vi "Load Patterns to Sessions.vi"(8 "error in":errorcluster, 10 "Pattern file paths":string[](array[string]), 11 "Sequence Context":refnum<k7>) -> (0 "error out":errorcluster)   [LabVIEW 2020, in "NIDigitalSPI.lvlib"]
uses:
  NIDigitalSPI.lvlib
  <vilib>/MeasurementLink/MeasurementLink Session Management Client/RPC Messages/ni_measurementlink_sessionmanagement_v1_ReserveSessionsRequest.ctl
  <vilib>/MeasurementLink/MeasurementLink Session Management Client/RPC Messages/ni_measurementlink_PinMapContext.ctl
  <vilib>/MeasurementLink/MeasurementLink Discovery Client/RPC Messages/ni_measurementlink_discovery_v1_ResolveServiceRequest.ctl
  <instrlib>/niDigital/niDigital.llb/niDigital gRPC Device Server.ctl
  <vilib>/MeasurementLink/MeasurementLink Session Management Client/MeasurementLink Session Management Client.lvlib
  <vilib>/MeasurementLink/MeasurementLink Discovery Client/MeasurementLink Discovery Client.lvlib
  <vilib>/MeasurementLink/MeasurementLink Measurement Server/MeasurementLink Measurement Server.lvlib
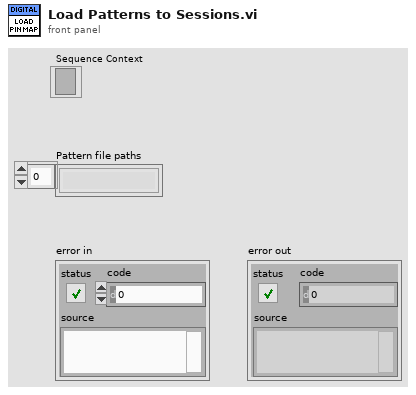
[diagram p1: front panel]
types:
  T1 = typedef "MeasurementLink Discovery Client.lvlib/ni_measurementlink_discovery_v1_ResolveServiceRequest.ctl" = cluster{"provided_interface":string, "service_class":string}
  T2 = typedef "MeasurementLink Session Management Client.lvlib/ni_measurementlink_sessionmanagement_v1_ReserveSessionsRequest.ctl" = cluster{"pin_map_context":T3, "pin_or_relay_names":string[], "instrument_type_id":string, "timeout_in_milliseconds":i32}
  T3 = typedef "MeasurementLink Session Management Client.lvlib/ni_measurementlink_PinMapContext.ctl" = cluster{"pin_map_id":string, "sites":i32[]}
  T4 = typedef "grpc-lvsupport-release.lvlib/grpcId.ctl" = u64
  T5 = typedef "MeasurementLink Discovery Client.lvlib/ni_measurementlink_discovery_v1_ServiceLocation.ctl" = cluster{"location":string, "insecure_port":string, "ssl_authenticated_port":string}
  T6 = typedef "MeasurementLink Session Management Client.lvlib/ni_measurementlink_sessionmanagement_v1_ReserveSessionsResponse.ctl" = cluster{"sessions":T7[]}
  T7 = typedef "MeasurementLink Session Management Client.lvlib/ni_measurementlink_sessionmanagement_v1_SessionInformation.ctl" = cluster{"session":T8, "resource_name":string, "channel_list":string, "instrument_type_id":string, "session_exists":bool, "channel_mappings":T9[]}
  T8 = typedef "MeasurementLink Session Management Client.lvlib/nidevice_grpc_Session.ctl" = cluster{"name":string}
  T9 = typedef "MeasurementLink Session Management Client.lvlib/ni_measurementlink_sessionmanagement_v1_ChannelMapping.ctl" = cluster{"pin_or_relay_name":string, "site":i32, "channel":string}
  T10 = typedef "niDigital gRPC Device Server.ctl" = cluster{"session name":string, "address (localhost)":string, "port (31763)":u32}
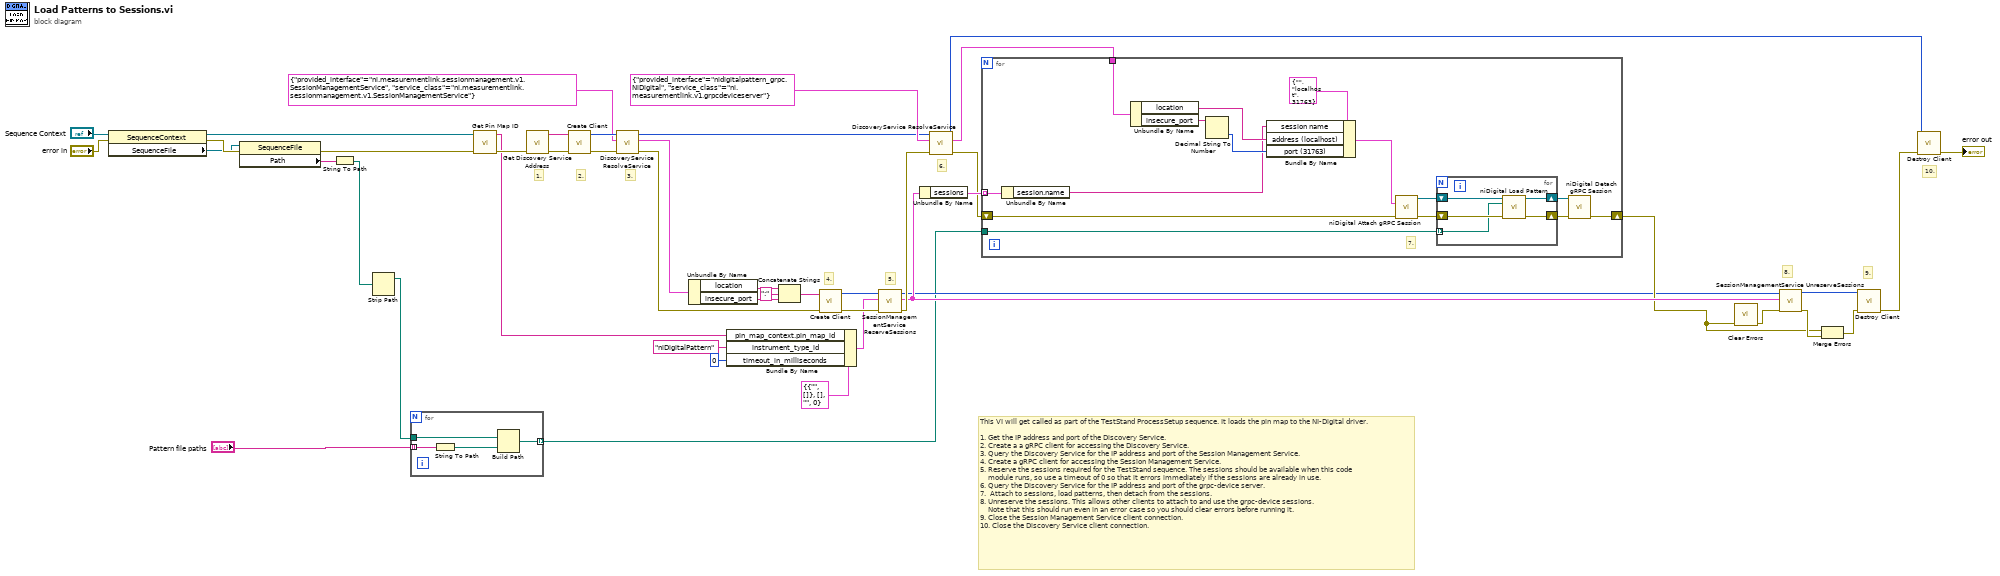
[diagram p0: block diagram]
diagram:
  # "10."
  # "9."
  # "8."
  # "6."
  # "5."
  # "4."
  # "3."
  # "2."
  # "1."
  # "This VI will get called as part of the TestStand ProcessSetup sequence. It loads the pin map to the NI-Digital driver.\n\n1. Get the IP address and port of the Discovery Service.\n2. Create a a gRPC client for accessing the Discovery Service.\n3. Query the Discovery Service for the IP address and port of the Session Management Service.\n4. Create a gRPC client for accessing the Session Management Service.\n5. Reserve the sessions required for the TestStand sequence. The sessions should be available when this code\n    module runs, so use a timeout of 0 so that it errors immediately if the sessions are already in use.  \n6. Query the Discovery Service for the IP address and port of the grpc-device server.\n7.  Attach to sessions, load patterns, then detach from the sessions.\n8. Unreserve the sessions. This allows other clients to attach to and use the grpc-device sessions. \n    Note that this should run even in an error case so you should clear errors before running it.\n9. Close the Session Management Service client connection.\n10. Close the Discovery Service client connection."
  n1 = property class="SequenceContext"(reference="Sequence Context", error in="error in") -> (reference out=w6:refnum<k7>, error out=w11:errorcluster, "SequenceFile"=w10:refnum<k7>)
  n2 = property class="SequenceFile"(reference=w10, error in=w11) -> (error out=w5:errorcluster, "Path"=w9:string)  [unwired: 1 out]
  n3 = String To Path(string=w9) -> (path=w4:path)
  n4 = Strip Path(path=w4) -> (stripped path=w2:path)  [unwired: 1 out]
  n5 = for {
    tunnel: "Pattern file paths" -> [w50] mode=indexing
    tunnel: [w47] -> w1 mode=indexing
    tunnel: w2 -> [w49]
    n6 = String To Path(string=w50) -> (path=w48:path)
    n7 = Build Path(base path=w49, name or relative path=w48) -> (appended path=w47:path)
  }
  n8 = call "Get Pin Map ID.vi"("error in"=w5, "Sequence Context"=w6) -> ("error out"=w20:errorcluster, "pin_map_id"=w19:string)  [unwired: 8 in]
  n9 = call <vilib>:"Get Discovery Service Address.vi"("error in"=w20) -> ("error out"=w27:errorcluster, "address"=w26:string)  [unwired: 9 in]
  n10 = call <vilib>:"Create Client.vi"("error in"=w27, "address"=w26) -> ("error out"=w43:errorcluster, "gRPC ID Out"=w44:T4)  [unwired: 8 in]
  n11 = call <vilib>:"DiscoveryService ResolveService.vi"("error in"=w43, "Request Data"=T1 {"provided_interface"="ni.measurementlink.sessionmanagement.v1.SessionManagementService", "service_class"="ni.measurementlink.sessionmanagement.v1.SessionManagementService"}, "gRPC ID"=w44) -> ("error out"=w42:errorcluster, "Response Data"=w14:T5, "gRPC ID out"=w33:T4)  [unwired: 6 in]
  n12 = Unbundle By Name(w14) -> ("location"=w16:string, "insecure_port"=w17:string)
  n13 = Bundle By Name(cluster=T2 {"pin_map_context"={"pin_map_id"="", "sites"=[]}, "pin_or_relay_names"=[], "instrument_type_id"="", "timeout_in_milliseconds"=0} ("Request Data"), "pin_map_context.pin_map_id"=w19, "instrument_type_id"="niDigitalPattern", "timeout_in_milliseconds"=0) -> (w38:T2)
  n14 = Concatenate Strings(w16, ":" ("string"), w17) -> (w15:string)
  n15 = call <vilib>:"Create Client.vi"("error in"=w42, "address"=w15) -> ("error out"=w45:errorcluster, "gRPC ID Out"=w46:T4)  [unwired: 8 in]
  n16 = call <vilib>:"SessionManagementService ReserveSessions.vi"("error in"=w45, "Request Data"=w38, "gRPC ID"=w46) -> ("error out"=w31:errorcluster, "Response Data"=w22:T6, "gRPC ID out"=w12:T4)  [unwired: 6 in]
  n17 = Unbundle By Name(w22) -> ("sessions"=w35:T7[])
  n18 = call <vilib>:"DiscoveryService ResolveService.vi"("error in"=w31, "Request Data"=T1 {"provided_interface"="nidigitalpattern_grpc.NiDigital", "service_class"="ni.measurementlink.v1.grpcdeviceserver"}, "gRPC ID"=w33) -> ("error out"=w30:errorcluster, "Response Data"=w29:T5, "gRPC ID out"=w32:T4)  [unwired: 6 in]
  n19 = for {
    tunnel: w35 -> [w64] mode=indexing
    shift-right: [w65] -> w13
    shift-left: w30 -> [w59]
    tunnel: w29 -> [w54]
    tunnel: w1 -> [w51]
    # "7."
    n20 = Unbundle By Name(w64) -> ("session.name"=w53:string)
    n21 = Unbundle By Name(w54) -> ("location"=w56:string, "insecure_port"=w57:string)
    n22 = Decimal String To Number(string=w57) -> (number=w58:i32)  [unwired: 2 in, 1 out]
    n23 = Bundle By Name(cluster=T10 {"session name"="", "address (localhost)"="localhost", "port (31763)"=31763} ("gRPC options"), "session name"=w53, "address (localhost)"=w56, "port (31763)"=w58) -> (w52:T10)
    n24 = call <instrlib>:"niDigital Attach gRPC Session.vi"("gRPC options"=w52, "error in"=w59) -> ("instrument handle out"=w60:refnum<k15>, "error out"=w61:errorcluster)  [unwired: 12 in]
    n25 = for {
      shift-right: [w70] -> w63
      shift-left: w61 -> [w68]
      shift-right: [w69] -> w62
      shift-left: w60 -> [w67]
      tunnel: w51 -> [w66] mode=indexing
      n26 = call <instrlib>:"niDigital Load Pattern.vi"("instrument handle"=w67, "pattern file"=w66, "error in"=w68) -> ("instrument handle out"=w69:refnum<k15>, "error out"=w70:errorcluster)  [unwired: 11 in]
    }
    n27 = call <instrlib>:"niDigital Detach gRPC Session.vi"("instrument handle"=w62, "error in"=w63) -> ("error out"=w65:errorcluster)  [unwired: 13 in]
  }
  n28 = call <vilib>:"Clear Errors.vi"("error in (no error)"=w13) -> ("error out"=w25:errorcluster)  [unwired: 5 in, 1 out]
  n29 = call <vilib>:"SessionManagementService UnreserveSessions.vi"("error in"=w25, "Request Data"=w22, "gRPC ID"=w12) -> ("error out"=w24:errorcluster, "gRPC ID out"=w36:T4)  [unwired: 6 in, 1 out]
  n30 = Merge Errors(w13, w24) -> (w23:errorcluster)
  n31 = call <vilib>:"Destroy Client.vi"("error in"=w23, "gRPC ID"=w36) -> ("error out"=w41:errorcluster)  [unwired: 9 in]
  n32 = call <vilib>:"Destroy Client.vi"("error in"=w41, "gRPC ID"=w32) -> ("error out"=→"error out":errorcluster)  [unwired: 9 in]
